vi "DiffDriveGetMaxSpeed.vi"() -> (3 "MaxSpeedFt/Sec":dbl)   [LabVIEW 2025]
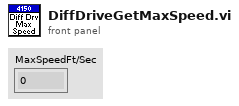
[diagram p1: front panel]
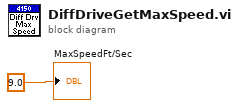
[diagram p0: block diagram]
diagram:
  "MaxSpeedFt/Sec" <- 9.0 ("MaxSpeedFt/Sec")
